vi "Sample--Sync_ExtClk_PXIe_PXI_PCIe_PCI.vi"() -> ()   [LabVIEW 2013]
doc: "This example demonstrates synchronizing two digitizers."
uses:
  <userlib>/ArtScope/Trigger/ArtScope_ConfigureTriggerDigital.vi
  <userlib>/ArtScope/Fetch/ArtScope_FetchBinary16.vi
  <userlib>/ArtScope/_SubVI/ArtScope_ArrayByChannel_U16.vi
panel:
  in  "reference position2":dbl
  in  "reference position":dbl
  in  "range(Vpp) 2":i32(ring) items=["20V", "10V", "2V", "40V", "16V", "8V", "4V", "1.6V", "800m", "400m", "160m", "80m", "40m"]
  in  "range(Vpp)":i32(ring) items=["20V", "10V", "2V", "40V", "16V", "8V", "4V", "1.6V", "800m", "400m", "160m", "80m", "40m"]
  in  "Slave":string="Dev2"
  in  "Master":string="Dev1"
  in  "Stop":bool
  out "Data2":u16[][](graph)
  in  "Timeout(s) 2":dbl=1.0
  in  "MinSampleRate 2":dbl=8000000.0
  in  "MinRecordLength2":i32=6000
  out "Data":u16[][](graph)
  out "ErrorOutput":errorcluster
  in  "Timeout(s)":dbl=1.0
  in  "MinRecordLength":i32=6000
  in  "MinSampleRate":dbl=8000000.0
  # "Vertical"
  # "Horizontal"
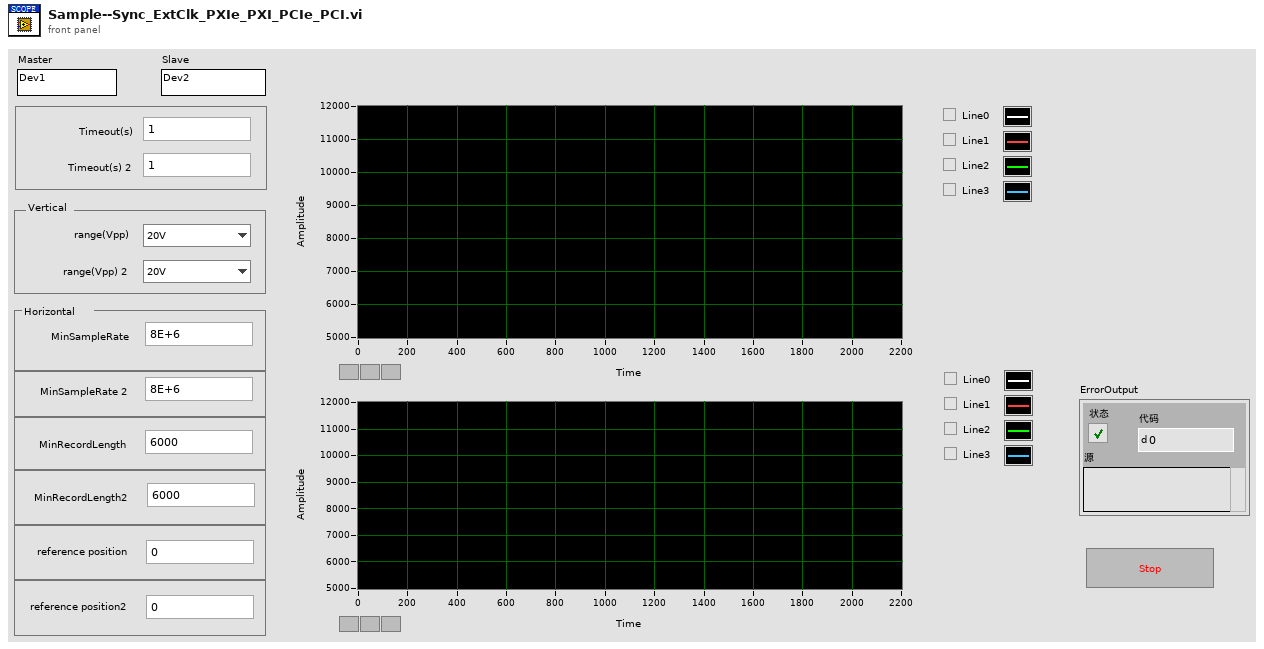
[diagram p1: front panel]
types:
  T1 = cluster{"fLSB":cluster{dbl, dbl, dbl, dbl, dbl, dbl, dbl, dbl}, "RangeValue":cluster{dbl, dbl, dbl, dbl, dbl, dbl, dbl, dbl}, "wMaxLSB":u32, "TriggerMode":i32, "sampLengthPerChan":u32, "pAvailSampsPoints":u32, "channelCount":i32}
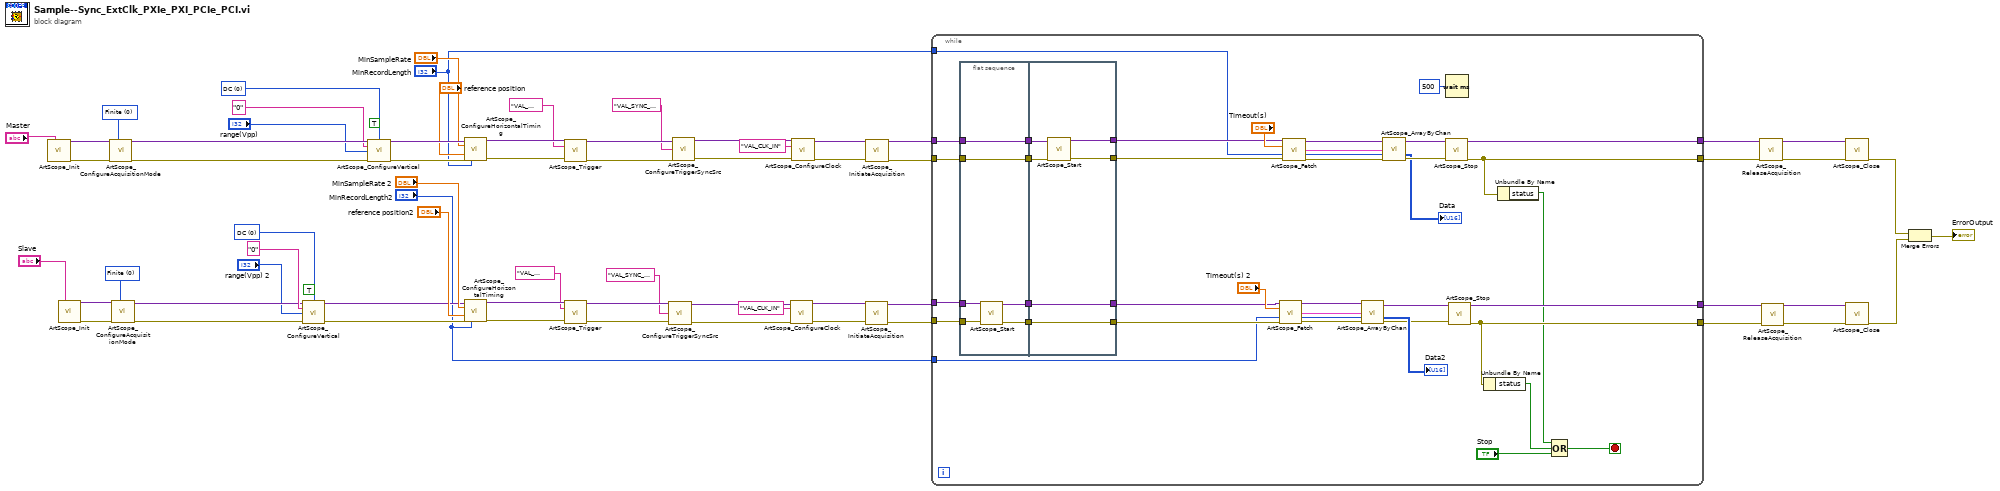
[diagram p0: block diagram]
diagram:
  (unwired) TRUE ("Enable")
  (unwired) TRUE ("Enable")
  w44 = 0 items=["DC", "AC"] ("Coupling")
  w52 = 0 items=["Finite", "Continuous"] ("AcuqMode")
  w62 = 0 items=["DC", "AC"] ("Coupling")
  w57 = 0 items=["Finite", "Continuous"] ("AcuqMode")
  n1 = call <userlib>:"ArtScope_Init.vi"("task name"="Master") -> ("task handle"=w39:variant, "error out"=w38:errorcluster)  [unwired: 13 in]
  n2 = call <userlib>:"ArtScope_Init.vi"("task name"="Slave") -> ("task handle"=w36:variant, "error out"=w35:errorcluster)  [unwired: 13 in]
  n3 = call <userlib>:"ArtScope_ConfigureAcquisitionMode.vi"("task handle"=w39, "acquisition mode"=w57, "error in (no error)"=w38) -> ("task handle"=w56:variant, "error out"=w58:errorcluster)  [unwired: 11 in]
  n4 = call <userlib>:"ArtScope_ConfigureAcquisitionMode.vi"("task handle"=w36, "acquisition mode"=w52, "error in (no error)"=w35) -> ("task handle"=w43:variant, "error out"=w42:errorcluster)  [unwired: 11 in]
  n5 = call <userlib>:"ArtScope_ConfigureVertical.vi"("task handle"=w43, "coupling"=w44, "channels"="0" ("Channel Name"), "range(Vpp)"="range(Vpp) 2", "error in (no error)"=w42) -> ("task handle"=w45:variant, "error out"=w46:errorcluster)  [unwired: 9 in]
  n6 = call <userlib>:"ArtScope_ConfigureVertical.vi"("task handle"=w56, "coupling"=w62, "channels"="0" ("Channel Name"), "range(Vpp)"="range(Vpp)", "error in (no error)"=w58) -> ("task handle"=w61:variant, "error out"=w60:errorcluster)  [unwired: 9 in]
  n7 = call <userlib>:"ArtScope_ConfigureHorizontalTiming.vi"("task handle"=w61, "min sample rate"="MinSampleRate", "reference position"="reference position", "error in (no error)"=w60, "min record length"="MinRecordLength") -> ("task handle"=w41:variant, "error out"=w55:errorcluster)  [unwired: 9 in]
  n8 = call <userlib>:"ArtScope_ConfigureHorizontalTiming.vi"("task handle"=w45, "min sample rate"="MinSampleRate 2", "reference position"="reference position2", "error in (no error)"=w46, "min record length"="MinRecordLength2") -> ("task handle"=w49:variant, "error out"=w48:errorcluster)  [unwired: 9 in]
  n9 = call-poly <userlib>:"ArtScope_Trigger.vi"("task handle"=w41, "trigger source"="VAL_TRIGGER_DTR", "error in"=w55) -> ("task handle"=w12:variant, "error out"=w10:errorcluster)  [unwired: 11 in]
  n10 = call-poly <userlib>:"ArtScope_Trigger.vi"("task handle"=w49, "trigger source"="VAL_TRIGGER_SYNCTRIGGER" ("TriggerSource"), "error in"=w48) -> ("task handle"=w7:variant, "error out"=w5:errorcluster)  [unwired: 11 in]
  n11 = call <userlib>:"ArtScope_ConfigureTriggerSyncSrc.vi"("task handle"=w7, "trigger sync source"="VAL_SYNC_TRIGGER0", "error in (no error)"=w5) -> ("task handle"=w6:variant, "error out"=w4:errorcluster)  [unwired: 11 in]
  n12 = call <userlib>:"ArtScope_ConfigureTriggerSyncSrc.vi"("task handle"=w12, "trigger sync source"="VAL_SYNC_TRIGGER0", "error in (no error)"=w10) -> ("task handle"=w11:variant, "error out"=w9:errorcluster)  [unwired: 11 in]
  n13 = call <userlib>:"ArtScope_ConfigureClock.vi"("task handle"=w6, "input clock source"="VAL_CLK_IN", "error in (no error)"=w4) -> ("task handle"=w33:variant, "error out"=w31:errorcluster)  [unwired: 11 in]
  n14 = call <userlib>:"ArtScope_ConfigureClock.vi"("task handle"=w11, "input clock source"="VAL_CLK_IN", "error in (no error)"=w9) -> ("task handle"=w27:variant, "error out"=w29:errorcluster)  [unwired: 11 in]
  n15 = call <userlib>:"ArtScope_InitiateAcquisition.vi"("task handle"=w33, "error in (no error)"=w31) -> ("task handle"=w32:variant, "error out"=w30:errorcluster)  [unwired: 12 in]
  n16 = call <userlib>:"ArtScope_InitiateAcquisition.vi"("task handle"=w27, "error in (no error)"=w29) -> ("task handle"=w26:variant, "error out"=w28:errorcluster)  [unwired: 12 in]
  n17 = while {
    tunnel: [w102] -> w25
    tunnel: [w89] -> w23
    tunnel: [w91] -> w21
    tunnel: [w101] -> w18
    tunnel: w32 -> [w100]
    tunnel: w30 -> [w99]
    tunnel: w26 -> [w95]
    tunnel: w28 -> [w94]
    tunnel: "MinRecordLength" -> [w81]
    tunnel: "MinRecordLength2" -> [w80]
    stop <- w86 stop-if-true
    n18 = flat-sequence {
      tunnel: w100 -> [w110]
      tunnel: w99 -> [w109]
      tunnel: [w105] -> w104
      tunnel: [w108] -> w103
      tunnel: [w107] -> w96
      tunnel: w95 -> [w107]
      tunnel: w94 -> [w106]
      tunnel: [w106] -> w93
      tunnel: w104 -> [w116]
      tunnel: w103 -> [w115]
      tunnel: w96 -> [w114]
      tunnel: w93 -> [w113]
      tunnel: [w116] -> w85
      tunnel: [w115] -> w84
      tunnel: [w112] -> w83
      tunnel: [w111] -> w82
      frame #0 {
        n19 = call <userlib>:"ArtScope_Start.vi"("task handle"=w110, "error in (no error)"=w109) -> ("task handle"=w105:variant, "error out"=w108:errorcluster)  [unwired: 12 in]
      }
      frame #1 {
        n20 = call <userlib>:"ArtScope_Start.vi"("task handle"=w114, "error in (no error)"=w113) -> ("task handle"=w112:variant, "error out"=w111:errorcluster)  [unwired: 12 in]
      }
    }
    n21 = call-poly <userlib>:"ArtScope_Fetch.vi"("task handle"=w85, "timeout"="Timeout(s) 2", "num samples"=w80, "error in (no error)"=w84) -> ("task handle"=w69:variant, "wfm info"=w67:T1, "data"=w66:u16[], "error out"=w68:errorcluster)  [unwired: 8 in]
    n22 = call-poly <userlib>:"ArtScope_Fetch.vi"("task handle"=w83, "timeout"="Timeout(s)", "num samples"=w81, "error in (no error)"=w82) -> ("task handle"=w79:variant, "wfm info"=w74:T1, "data"=w73:u16[], "error out"=w78:errorcluster)  [unwired: 8 in]
    n23 = call-poly <userlib>:"ArtScope_ArrayByChan.vi"("task handle"=w69, "wfm info"=w67, "1D data"=w66, "error in (no error)"=w68) -> ("task handle"=w70:variant, "2D data"=→"Data2":u16[][], "error out"=w71:errorcluster)  [unwired: 9 in]
    n24 = call-poly <userlib>:"ArtScope_ArrayByChan.vi"("task handle"=w79, "wfm info"=w74, "1D data"=w73, "error in (no error)"=w78) -> ("task handle"=w76:variant, "2D data"=→"Data":u16[][], "error out"=w77:errorcluster)  [unwired: 9 in]
    n25 = call <userlib>:"ArtScope_Stop.vi"("task handle"=w76, "error in"=w77) -> ("task handle"=w102:variant, "error out"=w89:errorcluster)  [unwired: 12 in]
    n26 = Wait (ms)(milliseconds to wait=u32 500 ("等待时间（毫秒）")) -> ()  [unwired: 1 out]
    n27 = call <userlib>:"ArtScope_Stop.vi"("task handle"=w70, "error in"=w71) -> ("task handle"=w101:variant, "error out"=w91:errorcluster)  [unwired: 12 in]
    n28 = Unbundle By Name(w91) -> ("status"=w90:bool)
    n29 = Unbundle By Name(w89) -> ("status"=w88:bool)
    n30 = Compound Arithmetic op=OR(w88, w90, "Stop") -> (w86:bool)
  }
  n31 = call <userlib>:"ArtScope_ReleaseAcquisition.vi"("task handle"=w25, "error in (no error)"=w23) -> ("task handle"=w24:variant, "error out"=w22:errorcluster)  [unwired: 12 in]
  n32 = call <userlib>:"ArtScope_ReleaseAcquisition.vi"("task handle"=w18, "error in (no error)"=w21) -> ("task handle"=w19:variant, "error out"=w20:errorcluster)  [unwired: 12 in]
  n33 = call <userlib>:"ArtScope_Close.vi"("task handle"=w24, "error in (no error)"=w22) -> ("error out"=w65:errorcluster)  [unwired: 13 in]
  n34 = call <userlib>:"ArtScope_Close.vi"("task handle"=w19, "error in (no error)"=w20) -> ("error out"=w64:errorcluster)  [unwired: 13 in]
  n35 = Merge Errors(w65, w64) -> (→"ErrorOutput":errorcluster)
